vi "Exit Structure.vi"(0 "Diagram in":refnum<vi>, 5 "Outputs":refnum<vi>[](array[refnum]), 11 "error in (no error)":errorcluster) -> (4 "Diagram out":refnum<vi>, 6 "Outputs":refnum<vi>[](array[refnum]), 15 "error out":errorcluster)   [LabVIEW 2015, in "Scripting.lvlib"]
uses:
  Scripting.lvlib
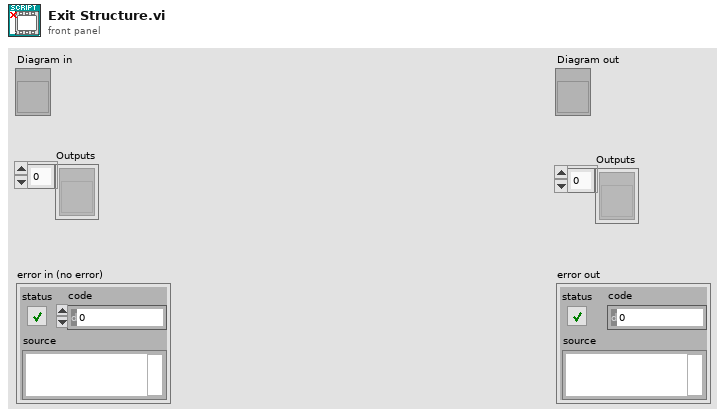
[diagram p1: front panel]
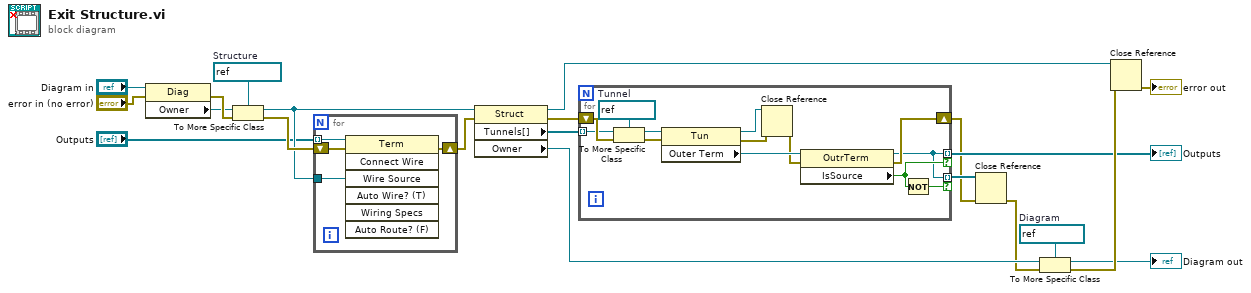
[diagram p0: block diagram]
diagram:
  w16 = refnum<vi> refnum  # Diagram
  w19 = refnum<vi> refnum  # Structure
  n1 = property class="Diag"(reference="Diagram in", error in="error in (no error)") -> (error out=w20:errorcluster, "Owner"=w18:refnum<vi>)  [unwired: 1 out]
  n2 = To More Specific Class(target class=w19, reference=w18, error in=w20) -> (specific class reference=w15:refnum<vi>, error out=w21:errorcluster)
  n3 = for {
    tunnel: w15 -> [w24]
    shift-right: [w23] -> w14
    shift-left: w21 -> [w25]
    tunnel: "Outputs" -> [w22] mode=indexing
    n4 = invoke class="Term" method="Connect Wire"(reference=w22, error in=w25, "Wire Source"=w24) -> (error out=w23:errorcluster)  [unwired: 4 in, 6 out]
  }
  n5 = property class="Struct"(reference=w15, error in=w14) -> (reference out=w4:refnum<vi>, error out=w5:errorcluster, "Tunnels[]"=w6:refnum<vi>[], "Owner"=w7:refnum<vi>)
  n6 = for {
    tunnel: w6 -> [w34] mode=indexing
    tunnel: [w27] -> w9 mode=indexing if=w28
    shift-right: [w36] -> w2
    shift-left: w5 -> [w38]
    tunnel: [w27] -> w3 mode=indexing if=w26
    w32 = refnum<vi> refnum  # Tunnel
    n7 = To More Specific Class(target class=w32, reference=w34, error in=w38) -> (specific class reference=w33:refnum<vi>, error out=w35:errorcluster)
    n8 = property class="Tun"(reference=w33, error in=w35) -> (reference out=w31:refnum<vi>, error out=w30:errorcluster, "Outer Term"=w37:refnum<vi>)
    n9 = Close Reference(reference=w31, error in (no error)=w30) -> (error out=w29:errorcluster)
    n10 = property class="OutrTerm"(reference=w37, error in=w29) -> (reference out=w27:refnum<vi>, error out=w36:errorcluster, "IsSource"=w28:bool)
    n11 = Not(x=w28) -> (.not. x?=w26:bool)
  }
  "Outputs" <- w9
  n12 = Close Reference(reference=w3, error in (no error)=w2) -> (error out=w1:errorcluster)
  n13 = To More Specific Class(target class=w16, reference=w7, error in=w1) -> (specific class reference=→"Diagram out":refnum<vi>, error out=w17:errorcluster)
  n14 = Close Reference(reference=w4, error in (no error)=w17) -> (error out=→"error out":errorcluster)
